vi "PathPlanner_Cmd_FollowLTVUnicyclePathPack.vi"(0 "Period":dbl=0.02, 1 "ControlPastEnd_Sec":dbl=3.0, 4 "Rotation Tolerance DEG":dbl=0.0872665, 5 "Trigger Events":bool=TRUE, 6 "Y Tolerance M":dbl=0.0762, 7 "ReplanningConfig":T16={"enableInitialReplanning"=TRUE, "enableDynamicReplanning"=FALSE, "dynamicReplanningTotalErrorThreshold"=1.0, "dynamicReplanningErrorSpikeThreshold"=0.25}, 8 "X Tolerance M":dbl=0.0762, 9 "Max Speed M/S":dbl=4.0, 10 "Track Width Meters":dbl=1.0, 11 "LTV_Unicycle_Ctrl_Model":T15={"Max linear ctrl effort M/S"=1.0, "Max angular ctrl effort Rad/S"=2.0, "Max Heading Meas Tol Rad"=0.2, "Max X Pos Meas Tol M"=0.0625, "Max Y Pos Meas Tol M"=0.125, "Max Linear Vel M/S"=9.0} {"Max Linear Vel M/S" format="%#_13g"; "Max Y Pos Meas Tol M" format="%#_13g"; "Max X Pos Meas Tol M" format="%#_13g"; "Max Heading Meas Tol Rad" format="%#_13g"; "Max angular ctrl effort Rad/S" format="%#_13g"; "Max linear ctrl effort M/S" format="%#_13g"}) -> (3 "PathPlanner_Ctrl_LTVUnicycleDrvConfig":T17={"ControlPastEnd_Sec"=3.0, "ReplanningConfig"={"enableInitialReplanning"=TRUE, "enableDynamicReplanning"=FALSE, "dynamicReplanningTotalErrorThreshold"=1.0, "dynamicReplanningErrorSpikeThreshold"=0.25}, "Trigger Events"=TRUE, "LTV_Unicycle_Ctrl_Model"={"Max linear ctrl effort M/S"=2.0, "Max angular ctrl effort Rad/S"=0.7, "Max Heading Meas Tol Rad"=2.0, "Max X Pos Meas Tol M"=0.7, "Max Y Pos Meas Tol M"=0.7, "Max Linear Vel M/S"=2.0}, "X Tolerance M"=2.0, "Y Tolerance M"=0.0762, "Rotation Tolerance DEG"=0.0872665, "Track Width Meters"=1.0, "Max Speed M/S"=4.0, "Period"=0.02} {"LTV_Unicycle_Ctrl_Model"."Max Linear Vel M/S" format="%#_13g"; "LTV_Unicycle_Ctrl_Model"."Max Y Pos Meas Tol M" format="%#_13g"; "LTV_Unicycle_Ctrl_Model"."Max X Pos Meas Tol M" format="%#_13g"; "LTV_Unicycle_Ctrl_Model"."Max Heading Meas Tol Rad" format="%#_13g"; "LTV_Unicycle_Ctrl_Model"."Max angular ctrl effort Rad/S" format="%#_13g"; "LTV_Unicycle_Ctrl_Model"."Max linear ctrl effort M/S" format="%#_13g"})   [LabVIEW 2019, in "PathPlanner24.lvlib"]
doc: "DOCUMENTATION IS NOT COMPLETE.\n \nPack controller tuning configuration for Path Planner Holonomic Drive Controller.\n\nInputs:\n - X PID Tuning - cluster - Input from PACK PROF PID VI\n - Y PID Tuning - cluster - Input from PACK PROF PID VI\n - thetaController - cluster - A profiled PID controller to respond to error in angle.\n - Max Wheel Speed M/.S - double - Maximum wheel speed (M/S)\n - DriveBaseRadius - double - The radius of the drive base in meters. For swerve drive, this is the\n distance from the center of the robot to the furthest module. For \n mecanum, this is the drive base width / 2\n - X Tolerance - double - X tolerance for calculating At Reference (Meters) (Optional. Default: 0.0762 )\n - Y Tolerance - double - Y tolerance for calculating At Reference (Meters) (Optional. Default: 0.0762 )\n - Rotation Tolerance - double - Rotation tolerance for calculating At Reference (Degrees) (Optional. Default: 0.0)873)\n\nOutputs:\n -- PathPlannerHolCtrlConfig -- cluster - packed controller configuration."
uses:
  PathPlanner24.lvlib
  TypeDef/PathPlannerCmdFollowLTVUnicycleConfig.ctl
  TypeDef/PathPlannerReplanningConfig.ctl
  <vilib>/Rock Robotics/WPI/ThirdParty/JAS_Junk/TrajLib/TypeDef/LTV_UNICYCLE_CONTROLLER_MODEL_PARAMS.CTL
  <vilib>/Rock Robotics/WPI/ThirdParty/JAS_Junk/TrajLib/Trajectory_Library.lvlib
  <vilib>/Rock Robotics/WPI/ThirdParty/JAS_Junk/TrajLib/TypeDef/ROTATION2D.ctl
  TypeDef/PathPlannerRotationTarget.ctl
  TypeDef/PathPlannerPathConstraints.ctl
  TypeDef/PathPlannerConstraintsZone.ctl
  ENum/PathPlanner_CommandUtilType_ENUM.ctl
  TypeDef/PathPlannerCommandUtil.ctl
  TypeDef/PathPlannerEventMarker.ctl
  TypeDef/PathPlannerGoalEndState.ctl
  <vilib>/Rock Robotics/WPI/ThirdParty/JAS_Junk/TrajLib/TypeDef/TRANSLATION2D.ctl
  TypeDef/PathPlannerPathPoint.ctl
  TypeDef/PathPlannerWaypoint.ctl
  TypeDef/PathPlannerPointTowardsZone.ctl
  TypeDef/PathPlannerIdealStartingState.ctl
  TypeDef/PathPlannerPath.ctl
panel:
  in  "PathPlannerPath":T1={"Reversed"=FALSE, "RotationTargets"=[], "ConstraintZones"=[], "EventMarkers"=[], "GlobalConstraints"={"MaxVelocityMps;"=0.0, "MaxAccelerationMpsSq;"=0.0, "MaxAngularVelRadPsEc;"=0.0, "MaxAngularAccRadPSecSq"=0.0, "Exists"=FALSE, "Unlimited"=FALSE, "NominalVoltageVolts"=12.0}, "GoalEndState"={"VelocityMPS"=0.0, "Rotation"={"VALUE"=0.0, "COS"=1.0, "SIN"=0.0}}, "AllPoints"=[], "Name"="", "Waypoints"=[], "PointTowardsZones"=[], "IdealStartingState"={"VelocityMPS"=0.0, "Rotation"={"VALUE"=1.0, "COS"=0.0, "SIN"=0.0}}, "IsChoreoPath"=FALSE, "PreventFlipping"=FALSE} {"IdealStartingState"."Rotation"."SIN" format="%13.4f"; "IdealStartingState"."Rotation"."COS" format="%13.4f"; "IdealStartingState"."Rotation"."VALUE" format="%13.4f"; "PointTowardsZones"."TargetPosition"."Y" format="%14.3f"; "PointTowardsZones"."TargetPosition"."X" format="%14.3f"; "PointTowardsZones"."RotationOffset"."SIN" format="%13.4f"; "PointTowardsZones"."RotationOffset"."COS" format="%13.4f"; "PointTowardsZones"."RotationOffset"."VALUE" format="%13.4f"; "Waypoints"."nextControl"."Y" format="%14.3f"; "Waypoints"."nextControl"."X" format="%14.3f"; "Waypoints"."anchor"."Y" format="%14.3f"; "Waypoints"."anchor"."X" format="%14.3f"; "Waypoints"."prevControl"."Y" format="%14.3f"; "Waypoints"."prevControl"."X" format="%14.3f"; "AllPoints"."RotationTarget"."rotation"."SIN" format="%13.4f"; "AllPoints"."RotationTarget"."rotation"."COS" format="%13.4f"; "AllPoints"."RotationTarget"."rotation"."VALUE" format="%13.4f"; "AllPoints"."Position"."Y" format="%14.3f"; "AllPoints"."Position"."X" format="%14.3f"; "GoalEndState"."Rotation"."SIN" format="%13.4f"; "GoalEndState"."Rotation"."COS" format="%13.4f"; "GoalEndState"."Rotation"."VALUE" format="%13.4f"; "RotationTargets"."rotation"."SIN" format="%13.4f"; "RotationTargets"."rotation"."COS" format="%13.4f"; "RotationTargets"."rotation"."VALUE" format="%13.4f"}
  # "3 inches"
  # "5 deg"
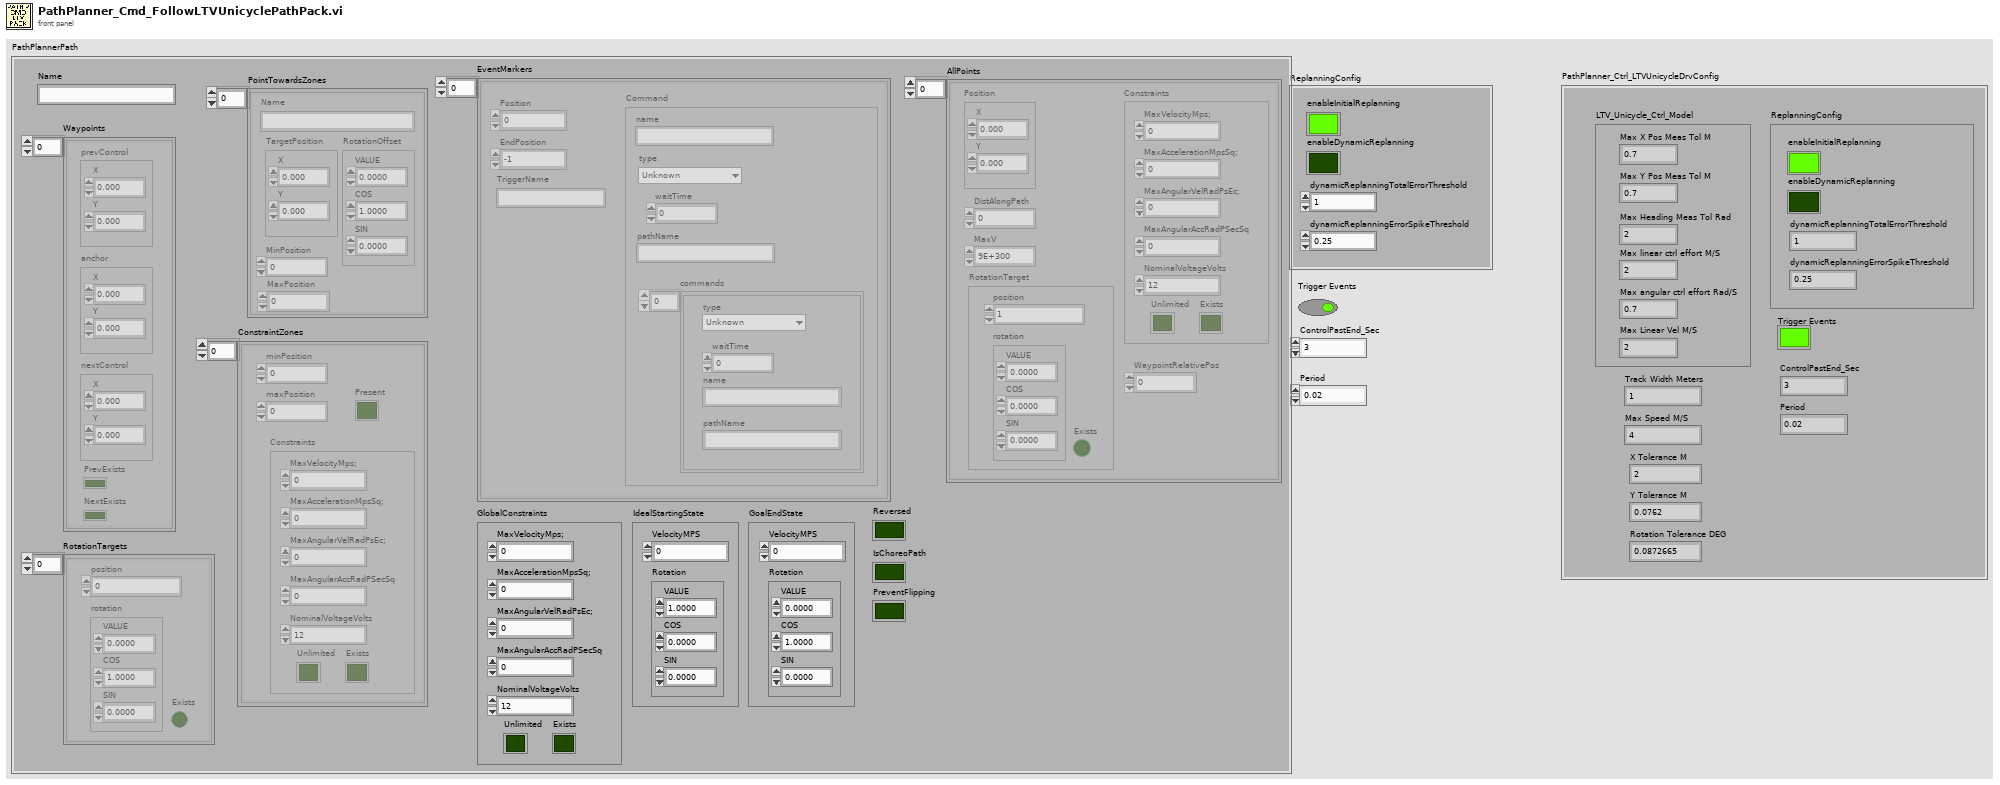
[diagram p1: front panel]
types:
  T1 = typedef "PathPlanner24.lvlib/PathPlannerPath.ctl" = cluster{"Reversed":bool, "RotationTargets":T2[], "ConstraintZones":T4[], "EventMarkers":T6[], "GlobalConstraints":T5, "GoalEndState":T9, "AllPoints":T10[], "Name":string, "Waypoints":T12[], "PointTowardsZones":T13[], "IdealStartingState":T14, "IsChoreoPath":bool, "PreventFlipping":bool}
  T2 = typedef "PathPlanner24.lvlib/PathPlannerRotationTarget.ctl" = cluster{"position":dbl, "rotation":T3, "Exists":bool}
  T3 = typedef "Trajectory_Library.lvlib/ROTATION2D.ctl" = cluster{"VALUE":dbl, "COS":dbl, "SIN":dbl}
  T4 = typedef "PathPlanner24.lvlib/PathPlannerConstraintsZone.ctl" = cluster{"minPosition":dbl, "maxPosition":dbl, "Constraints":T5, "Present":bool}
  T5 = typedef "PathPlanner24.lvlib/PathPlannerPathConstraints.ctl" = cluster{"MaxVelocityMps;":dbl, "MaxAccelerationMpsSq;":dbl, "MaxAngularVelRadPsEc;":dbl, "MaxAngularAccRadPSecSq":dbl, "Exists":bool, "Unlimited":bool, "NominalVoltageVolts":dbl}
  T6 = typedef "PathPlanner24.lvlib/PathPlannerEventMarker.ctl" = cluster{"Position":dbl, "Command":T7, "TriggerName":string, "EndPosition":dbl}
  T7 = typedef "PathPlanner24.lvlib/PathPlannerCommandUtil.ctl" = cluster{"waitTime":dbl, "name":string, "pathName":string, "commands":cluster{"type":T8, "waitTime":dbl, "name":string, "pathName":string}[], "type":T8}
  T8 = typedef "PathPlanner24.lvlib/PathPlanner_CommandUtilType_ENUM.ctl" = enum16{"Unknown", "Wait", "Named", "Path", "Sequential", "Parallel", "Race", "Deadline"}
  T9 = typedef "PathPlanner24.lvlib/PathPlannerGoalEndState.ctl" = cluster{"VelocityMPS":dbl, "Rotation":T3}
  T10 = typedef "PathPlanner24.lvlib/PathPlannerPathPoint.ctl" = cluster{"Position":T11, "DistAlongPath":dbl, "MaxV":dbl, "Constraints":T5, "RotationTarget":T2, "WaypointRelativePos":dbl}
  T11 = typedef "Trajectory_Library.lvlib/TRANSLATION2D.ctl" = cluster{"X":dbl, "Y":dbl}
  T12 = typedef "PathPlanner24.lvlib/PathPlannerWaypoint.ctl" = cluster{"prevControl":T11, "anchor":T11, "nextControl":T11, "PrevExists":bool, "NextExists":bool}
  T13 = typedef "PathPlanner24.lvlib/PathPlannerPointTowardsZone.ctl" = cluster{"RotationOffset":T3, "Name":string, "TargetPosition":T11, "MinPosition":dbl, "MaxPosition":dbl}
  T14 = typedef "PathPlanner24.lvlib/PathPlannerIdealStartingState.ctl" = cluster{"VelocityMPS":dbl, "Rotation":T3}
  T15 = typedef "Trajectory_Library.lvlib/LTV_UNICYCLE_CONTROLLER_MODEL_PARAMS.CTL" = cluster{"Max linear ctrl effort M/S":dbl, "Max angular ctrl effort Rad/S":dbl, "Max Heading Meas Tol Rad":dbl, "Max X Pos Meas Tol M":dbl, "Max Y Pos Meas Tol M":dbl, "Max Linear Vel M/S":dbl}
  T16 = typedef "PathPlanner24.lvlib/PathPlannerReplanningConfig.ctl" = cluster{"enableInitialReplanning":bool, "enableDynamicReplanning":bool, "dynamicReplanningTotalErrorThreshold":dbl, "dynamicReplanningErrorSpikeThreshold":dbl}
  T17 = typedef "PathPlanner24.lvlib/PathPlannerCmdFollowLTVUnicycleConfig.ctl" = cluster{"ControlPastEnd_Sec":dbl, "ReplanningConfig":T16, "Trigger Events":bool, "LTV_Unicycle_Ctrl_Model":T15, "X Tolerance M":dbl, "Y Tolerance M":dbl, "Rotation Tolerance DEG":dbl, "Track Width Meters":dbl, "Max Speed M/S":dbl, "Period":dbl}
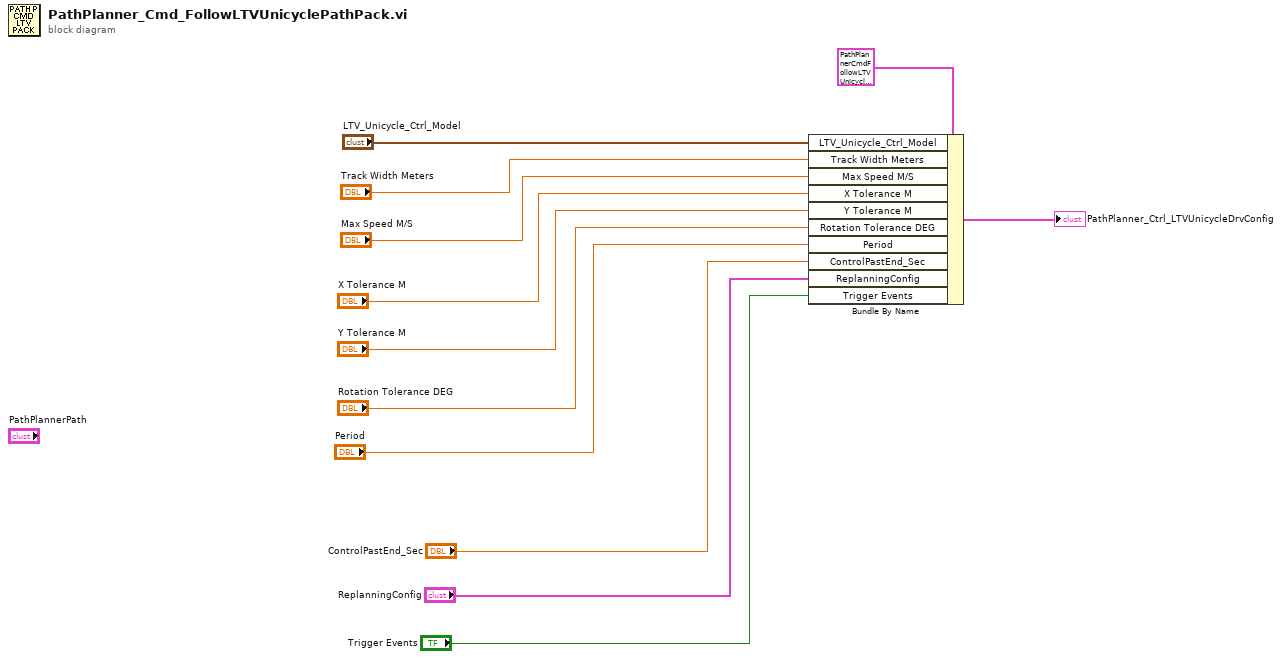
[diagram p0: block diagram]
diagram:
  n1 = Bundle By Name(cluster=T17 {"ControlPastEnd_Sec"=3.0, "ReplanningConfig"={"enableInitialReplanning"=TRUE, "enableDynamicReplanning"=FALSE, "dynamicReplanningTotalErrorThreshold"=1.0, "dynamicReplanningErrorSpikeThreshold"=0.25}, "Trigger Events"=TRUE, "LTV_Unicycle_Ctrl_Model"={"Max linear ctrl effort M/S"=2.0, "Max angular ctrl effort Rad/S"=0.7, "Max Heading Meas Tol Rad"=2.0, "Max X Pos Meas Tol M"=0.7, "Max Y Pos Meas Tol M"=0.7, "Max Linear Vel M/S"=2.0}, "X Tolerance M"=0.0762, "Y Tolerance M"=0.0762, "Rotation Tolerance DEG"=0.0872665, "Track Width Meters"=1.0, "Max Speed M/S"=4.0, "Period"=0.02} ("PathPlanner_Cmd_FollowLTVUnicycleConfig"), "LTV_Unicycle_Ctrl_Model"="LTV_Unicycle_Ctrl_Model", "Track Width Meters"="Track Width Meters", "Max Speed M/S"="Max Speed M/S", "X Tolerance M"="X Tolerance M", "Y Tolerance M"="Y Tolerance M", "Rotation Tolerance DEG"="Rotation Tolerance DEG", "Period"="Period", "ControlPastEnd_Sec"="ControlPastEnd_Sec", "ReplanningConfig"="ReplanningConfig", "Trigger Events"="Trigger Events") -> (→"PathPlanner_Ctrl_LTVUnicycleDrvConfig":T17)
